vi "interpolation and caculate mean (SubVI).vi"(0 "upper":dbl[](array[numeric]), 1 "upper time":dbl[](array[numeric]), 2 "lower":dbl[](array[numeric]), 3 "lower time":dbl[](array[numeric]), 4 "original":dbl[](array[numeric])) -> (5 "up+mean+low":dbl[][](array[numeric]), 6 "mean after interpolation":dbl[](array[numeric]), 7 "upper time afi":dbl[](array[numeric]) format="%_6g", 8 "upper after interpolation":dbl[](array[numeric]), 9 "lower time afi":dbl[](array[numeric]) format="%_6g", 10 "lower after interpolation":dbl[](array[numeric]))   [LabVIEW 2018]
uses:
  <vilib>/gmath/NI_Gmath.lvlib
panel:
  out "Array 2":dbl[](array[numeric])
  out "Array":dbl[](array[numeric])
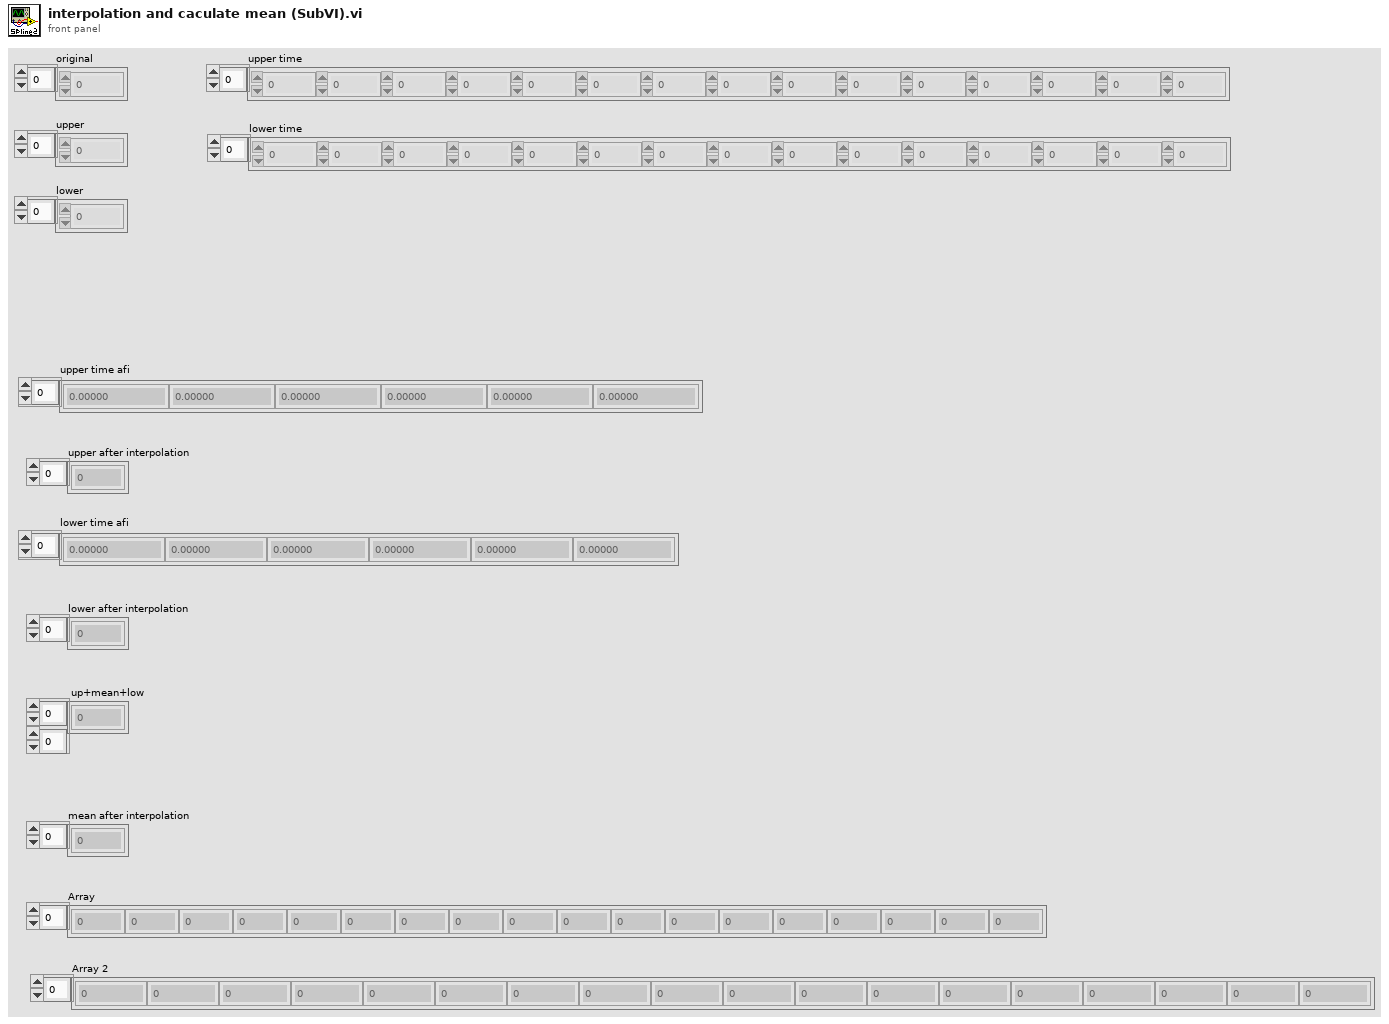
[diagram p1: front panel]
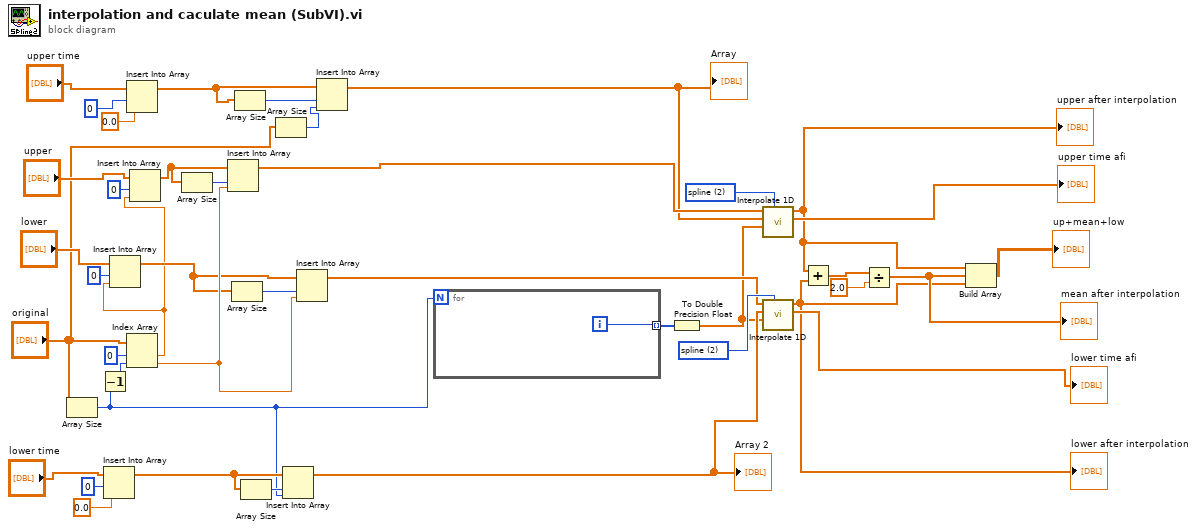
[diagram p0: block diagram]
diagram:
  w35 = 2 items=["nearest", "linear", "spline", "cubic Hermite", "Lagrange"] ("method")
  w34 = 2 items=["nearest", "linear", "spline", "cubic Hermite", "Lagrange"] ("method")
  n1 = Array Size(array="original") -> (size(s)=w4:i32)
  n2 = Decrement(x=w4) -> (x-1=w24:i32)
  n3 = Insert Into Array(array="lower time", index=0, new element=0.0 ("new element/subarray")) -> (w7:dbl[])
  n4 = Insert Into Array(array="upper time", index=0, new element=0.0 ("new element/subarray")) -> (w8:dbl[])
  n5 = Index Array(array="original", index #1=0 ("index"), index #2=w24) -> (element #1=w20:dbl, element #2=w25:dbl)
  n6 = Insert Into Array(array="lower", index=0, new element=w20) -> (w22:dbl[])
  n7 = Insert Into Array(array="upper", index=0, new element=w20) -> (w26:dbl[])
  n8 = Array Size(array=w26) -> (size(s)=w23:i32)
  n9 = Insert Into Array(array=w26, index=w23, new element=w25) -> (w19:dbl[])
  n10 = Array Size(array=w22) -> (size(s)=w28:i32)
  n11 = Array Size(array=w8) -> (size(s)=w14:i32)
  n12 = Array Size(array=w7) -> (size(s)=w11:i32)
  n13 = Array Size(array="original") -> (size(s)=w5:i32)
  n14 = Insert Into Array(array=w7, index=w11, new element=w4) -> (w3:dbl[])
  "Array 2" <- w3
  n15 = Insert Into Array(array=w22, index=w28, new element=w25) -> (w31:dbl[])
  n16 = Insert Into Array(array=w8, index=w14, new element=w5) -> (w2:dbl[])
  "Array" <- w2
  n17 = for {
    N: w4 -> [_]
    tunnel: [w42] -> w40 mode=indexing
    i -> [w42]
  }
  n18 = To Double Precision Float(number=w40) -> (double precision float=w1:dbl[])
  n19 = call <vilib>:"Interpolate 1D.vi"("method"=w34, "xi"=w1, "X"=w2, "Y"=w19) -> ("xi used"=→"upper time afi":dbl[], "yi"=w17:dbl[])  [unwired: 5 in, 1 out]
  "upper after interpolation" <- w17
  n20 = call <vilib>:"Interpolate 1D.vi"("method"=w35, "xi"=w1, "X"=w3, "Y"=w31) -> ("xi used"=→"lower time afi":dbl[], "yi"=w29:dbl[])  [unwired: 5 in, 1 out]
  "lower after interpolation" <- w29
  n21 = Add(x=w17, y=w29) -> (x+y=w37:dbl[])
  n22 = Divide(x=w37, y=2.0) -> (x/y=w41:dbl[])
  "mean after interpolation" <- w41
  n23 = Build Array(w17, w41, w29) -> (→"up+mean+low":dbl[][])
